vi "FP_QTMTelegram_MakeArray.vi"(7 "Array\nSize":i32=22, 11 "Data Frame":T1={"Timestamp"=115, "Framenumber"=28, "ComponentCount"=1, "Components"=[{"ComponentSize"=64, "ComponentType"=6, "Count"=1, "Padding"=0, "Data"=[[1.0], [3.0], [5.0], [7.0], [9.0], [11.0]]}]} {"Components"."ComponentType" items=["3D"=1, "3DRes"=9, "3DnoLabels"=2, "Analog"=3, "3DnoLabelsRes"=10, "Force"=4, "6D"=5, "6DRes"=11, "6DEuler"=6, "6DEulerRes"=12, "2D"=7, "2DLin"=8]}) -> (2 "NaN?":bool, 3 "ArrayOut":dbl[](array[numeric]))   [LabVIEW 2013]
uses:
  QTM Data Frame.ctl
  QTM ComonentType.ctl
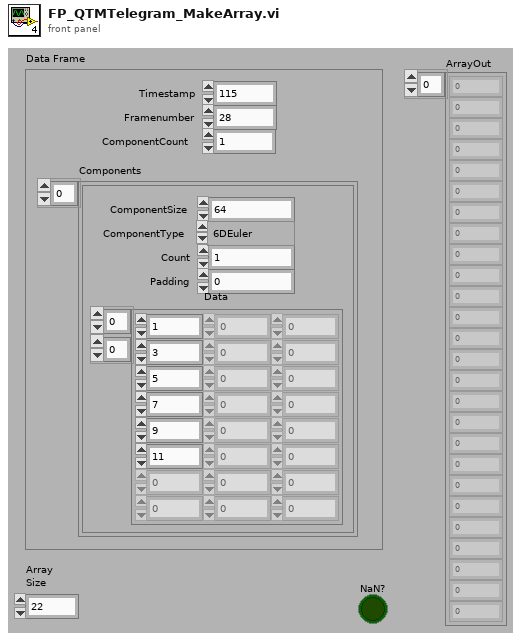
[diagram p1: front panel]
types:
  T1 = typedef "QTM Data Frame.ctl" = cluster{"Timestamp":i64, "Framenumber":i32, "ComponentCount":i32, "Components":cluster{"ComponentSize":i32, "ComponentType":T2, "Count":i32, "Padding":i32, "Data":dbl[][]}[]}
  T2 = typedef "QTM ComonentType.ctl" = i32
  T3 = cluster{"ComponentSize":i32, "ComponentType":T2, "Count":i32, "Padding":i32, "Data":dbl[][]}[]
  T4 = cluster{"ComponentSize":i32, "ComponentType":T2, "Count":i32, "Padding":i32, "Data":dbl[][]}
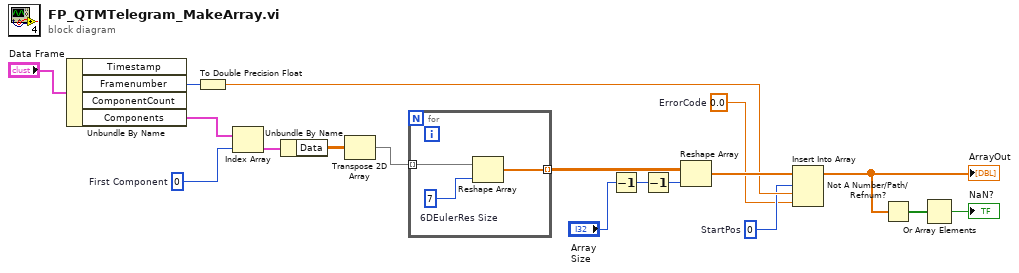
[diagram p0: block diagram]
diagram:
  w2 = 0.0  # ErrorCode
  w5 = 0  # StartPos
  w11 = 0  # First Component
  n1 = Unbundle By Name("Data Frame") -> ("Framenumber"=w17:i32, "Components"=w13:T3)  [unwired: 2 out]
  n2 = To Double Precision Float(number=w17) -> (double precision float=w6:dbl)
  n3 = Index Array(array=w13, index=w11) -> (element=w12:T4)
  n4 = Unbundle By Name(w12) -> ("Data"=w10:dbl[][])
  n5 = Transpose 2D Array(2D array=w10) -> (transposed array=w9:dbl[][])
  n6 = for {
    tunnel: [w19] -> w3 mode=indexing
    tunnel: w9 -> [w20] mode=indexing
    w21 = 7  # 6DEulerRes Size
    n7 = Reshape Array(w20, w21) -> (w19:dbl[])
  }
  n8 = Decrement(x="Array\nSize") -> (x-1=w8:i32)
  n9 = Decrement(x=w8) -> (x-1=w1:i32)
  n10 = Reshape Array(w3, w1) -> (w7:dbl[])
  n11 = Insert Into Array(array=w7, index=w5, new element #1=w6, new element #2=w2) -> (w4:dbl[])
  "ArrayOut" <- w4
  n12 = Not A Number/Path/Refnum?(number/path/refnum=w4) -> (NaN/Path/Refnum?=w15:bool[])
  n13 = Or Array Elements(Boolean array=w15) -> (logical OR=→"NaN?":bool)
